vi "Convert to Optimizer Interface State.vi"(8 "error in (no error)":errorcluster, 11 "Optimizer State in":T2) -> (0 "error out":errorcluster, 3 "Optimizer State out":variant)   [LabVIEW 2020, in "SQSnobFit Control Panel.lvlib" / "Remote Connection Manager.lvlib"]
doc: "Converts the internal optimizer state to a variant with attributes corresponding to fields needed by the remote system."
uses:
  Remote Connection Manager.lvlib
  Instrument Manager/Instrument State.ctl
  <vilib>/addons/zeromq/zmq_context.lvclass
  <vilib>/addons/zeromq/zmq_socket.lvclass
  Typedefs/Remote Optimizer State.ctl
  SQSnobFit Control Panel.lvlib
  Instrument Manager/Instrument Manager.lvlib
panel:
  out "Generic Optimizer State":T1
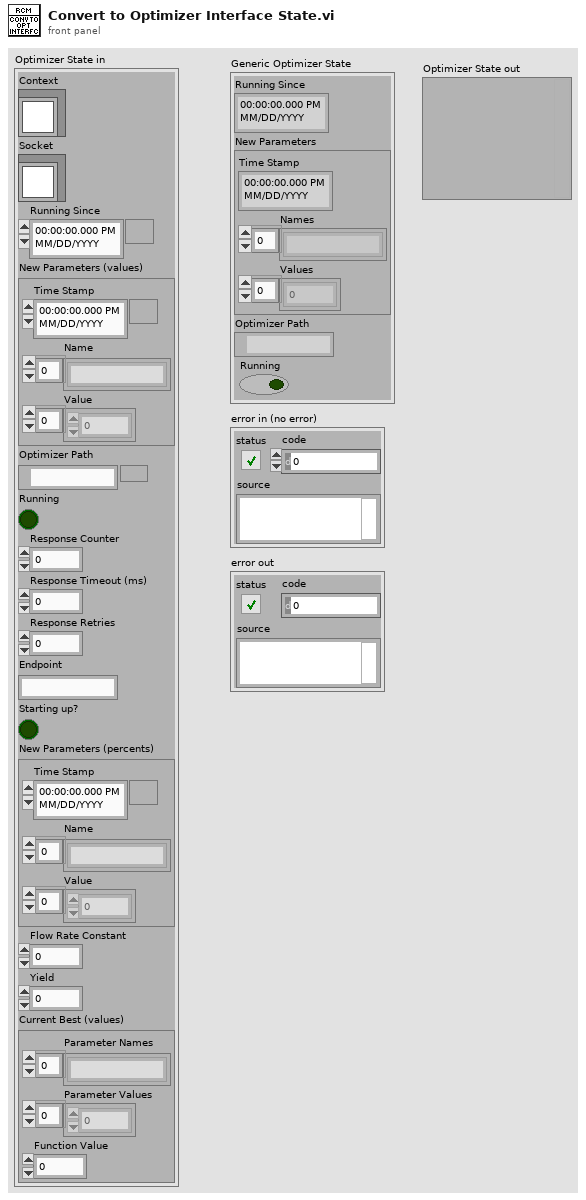
[diagram p1: front panel]
types:
  T1 = typedef "SQSnobFit Control Panel.lvlib/Remote Optimizer State.ctl" = cluster{"Running Since":timestamp, "New Parameters":cluster{"Time Stamp":timestamp, "Names":string[], "Values":dbl[]}, "Optimizer Path":path, "Running":bool}
  T2 = typedef "SQSnobFit Control Panel.lvlib/Instrument Manager.lvlib/Instrument State.ctl" = cluster{"Context":refnum<class "zmq_context.lvclass">, "Socket":refnum<class "zmq_socket.lvclass">, "Running Since":timestamp, "New Parameters (values)":cluster{"Time Stamp":timestamp, "Name":string[], "Value":dbl[]}, "Optimizer Path":path, "Running":bool, "Response Counter":u8, "Response Timeout (ms)":u32, "Response Retries":u32, "Endpoint":string, "Starting up?":bool, "New Parameters (percents)":cluster{"Time Stamp":timestamp, "Name":string[], "Value":dbl[]}, "Flow Rate Constant":dbl, "Yield":dbl, "Current Best (values)":cluster{"Parameter Names":string[], "Parameter Values":dbl[], "Function Value":dbl}}
  T3 = cluster{"Time Stamp":timestamp, "Name":string[], "Value":dbl[]}
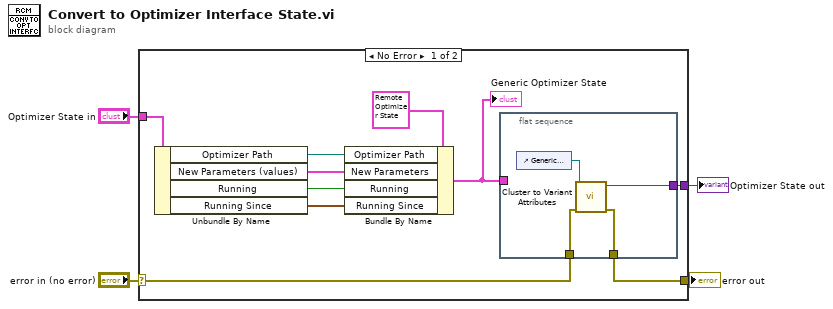
[diagram p0: block diagram]
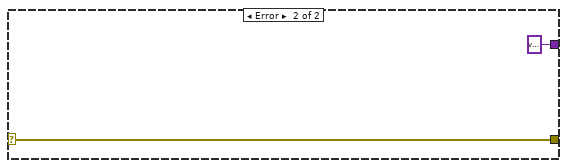
[diagram p2: hidden frame]
diagram:
  n1 = case shown="No Error" "error in (no error)" {
    selector: "error in (no error)" -> [w7 w20]
    tunnel: "Optimizer State in" -> [w14 _]
    tunnel: [w6 w20] -> w2
    tunnel: [w5 variant ("Variant out")] -> w1
    frame No Error {
      n2 = Unbundle By Name(w14) -> ("Optimizer Path"=w9:path, "New Parameters (values)"=w12:T3, "Running"=w10:bool, "Running Since"=w11:timestamp)
      n3 = Bundle By Name(cluster=T1 {"Running Since"=timestamp(0 s since 1904-01-01), "New Parameters"={"Time Stamp"=timestamp(0 s since 1904-01-01), "Names"=[], "Values"=[]}, "Optimizer Path"=path "", "Running"=FALSE} ("Generic Optimizer State"), "Optimizer Path"=w9, "New Parameters"=w12, "Running"=w10, "Running Since"=w11) -> (w8:T1)
      "Generic Optimizer State" <- w8
      n4 = flat-sequence {
        tunnel: w8 -> [_]
        tunnel: w7 -> [w17]
        tunnel: [w16] -> w6
        tunnel: [w15] -> w5
        frame #0 {
          n5 = control-ref of="Generic Optimizer State"() -> (w18:refnum<vi>)
          n6 = call "Cluster to Variant Attributes.vi"("error in (no error)"=w17, "Cluster in"=w18) -> ("error out"=w16:errorcluster, "Variant out"=w15:variant)  [unwired: 8 in]
        }
      }
    }
    frame Error {
    }
  }
  "error out" <- w2
  "Optimizer State out" <- w1
